vi "AIT 1553 System Definition API Example.vi"() -> ()   [LabVIEW 2011]
uses:
  Controls/AIT 1553 Settings.ctl
  System Explorer/Controls/1553 Bus Enabled.ctl
  NationalInstruments.VeriStand.SystemDefinitionAPI
  AIT 1553 Custom Device.lvlib
panel:
  out "error":string
  out "error out":errorcluster
  in  "error in (no error)":errorcluster
  out "Sysdef Path":path=path "C:/Users/Public/Documents/National Instruments/NI VeriStand 2011/Projects/DynamicallyCreatedProject/DynamicallyCreatedProject.nivssdf"
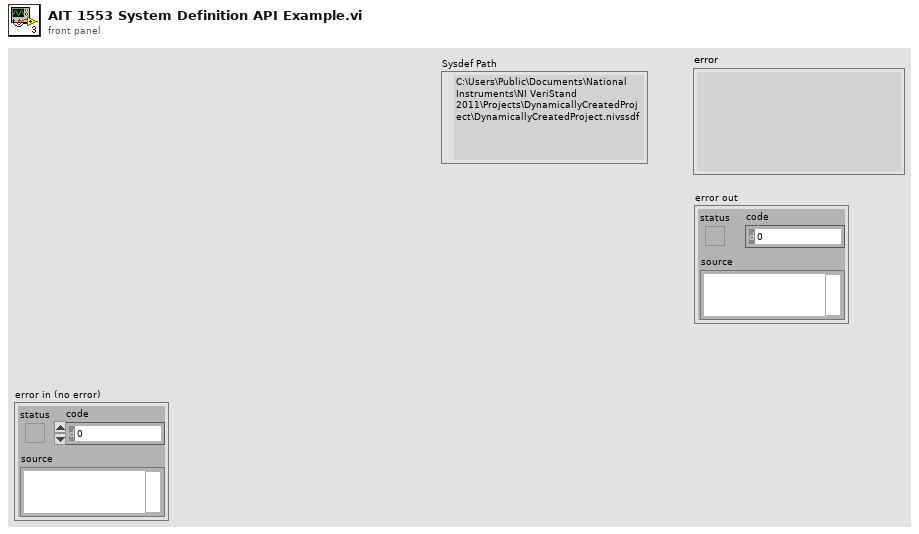
[diagram p1: front panel]
types:
  T1 = typedef "AIT 1553 Settings.ctl" = cluster{"Board Serial #":u64, "AppLicense":bool, "License Key":string, "BusEnabledProperties":T2, "Description":string, "Bus1 Path":path, "Bus2 Path":path, "Bus3 Path":path, "Bus4 Path":path}
  T2 = typedef "AIT 1553 Custom Device.lvlib/1553 Bus Enabled.ctl" = cluster{"Bus1Enabled":bool, "Bus2Enabled":bool, "Bus3Enabled":bool, "Bus4Enabled":bool}
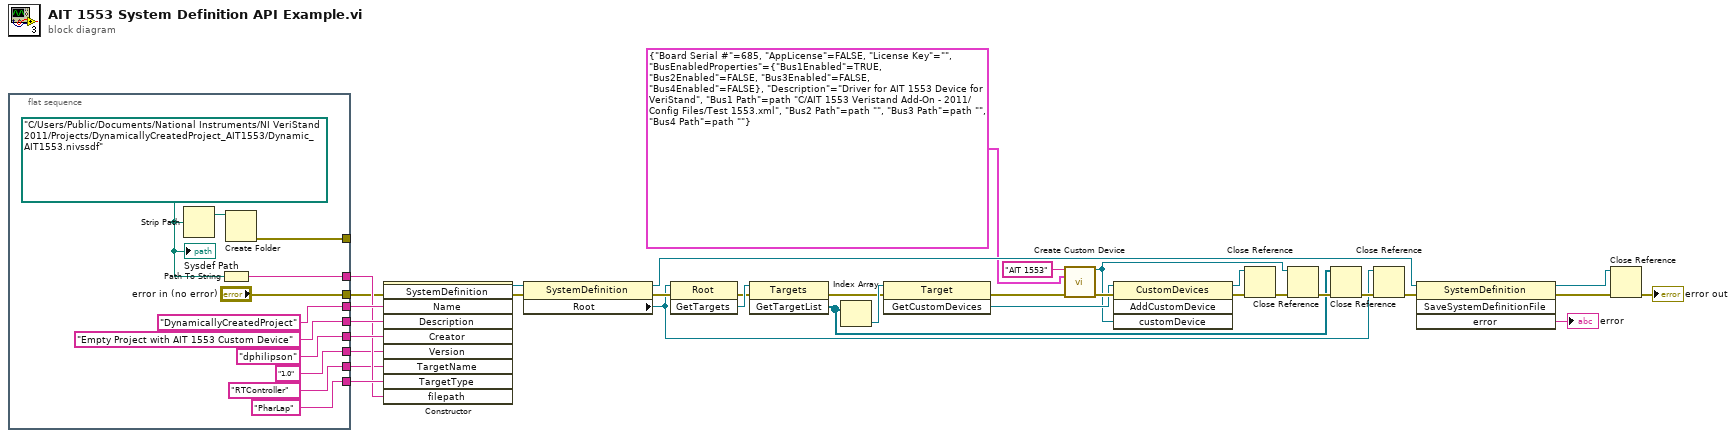
[diagram p0: block diagram]
diagram:
  n1 = flat-sequence {
    tunnel: ["DynamicallyCreatedProject" ("Name")] -> w34
    tunnel: ["dphilipson" ("Creator")] -> w33
    tunnel: ["RTController" ("TargetName")] -> w23
    tunnel: ["PharLap" ("TargetType")] -> w32
    tunnel: ["Empty Project with AIT 1553 Custom Device" ("Description")] -> w31
    tunnel: [w38] -> w30
    tunnel: [w37] -> _
    tunnel: ["error in (no error)"] -> w24
    tunnel: ["1.0" ("Version")] -> w22
    frame #0 {
      w39 = path "C:/Users/Public/Documents/National Instruments/NI VeriStand 2011/Projects/DynamicallyCreatedProject_AIT1553/Dynamic_AIT1553.nivssdf"
      n2 = Strip Path(path=w39) -> (stripped path=w40:path)  [unwired: 1 out]
      n3 = Path To String(path=w39) -> (string=w38:string)
      n4 = Create Folder(path (use dialog)=w40) -> (error out=w37:errorcluster)  [unwired: 2 in, 2 out]
      "Sysdef Path" <- w39
    }
  }
  n5 = constructor class="SystemDefinition"(error in=w24, "Name"=w34, "Description"=w31, "Creator"=w33, "Version"=w22, "TargetName"=w23, "TargetType"=w32, "filepath"=w30) -> (reference out=w26:refnum<k24>, error out=w28:errorcluster)  [unwired: 2 in, 8 out]
  n6 = property class="SystemDefinition"(reference=w26, error in=w28) -> (reference out=w13:refnum<k24>, error out=w27:errorcluster, "Root"=w12:refnum<k24>)
  n7 = invoke class="Root" method="GetTargets"(reference=w12, error in=w27) -> (error out=w25:errorcluster, "GetTargets"=w29:refnum<k24>)  [unwired: 1 in, 1 out]
  n8 = invoke class="Targets" method="GetTargetList"(reference=w29, error in=w25) -> (error out=w14:errorcluster, "GetTargetList"=w11:refnum<k24>[])  [unwired: 1 in, 1 out]
  n9 = Index Array(array=w11) -> (element=w15:refnum<k24>)  [unwired: 1 in]
  n10 = invoke class="Target" method="GetCustomDevices"(reference=w15, error in=w14) -> (error out=w10:errorcluster, "GetCustomDevices"=w5:refnum<k24>)  [unwired: 1 in, 1 out]
  n11 = call "Create Custom Device.vi"("Name"="AIT 1553", "AIT 1553 Settings"=T1 {"Board Serial #"=685, "AppLicense"=FALSE, "License Key"="", "BusEnabledProperties"={"Bus1Enabled"=TRUE, "Bus2Enabled"=FALSE, "Bus3Enabled"=FALSE, "Bus4Enabled"=FALSE}, "Description"="Driver for AIT 1553 Device for VeriStand", "Bus1 Path"=path "C:/AIT 1553 Veristand Add-On - 2011/Config Files/Test 1553.xml", "Bus2 Path"=path "", "Bus3 Path"=path "", "Bus4 Path"=path ""}, "error in (no error)"=w10) -> ("Custom Device reference"=w1:refnum<k24>, "error out"=w9:errorcluster)  [unwired: 11 in]
  n12 = invoke class="CustomDevices" method="AddCustomDevice"(reference=w5, error in=w9, "customDevice"=w1) -> (reference out=w4:refnum<k24>, error out=w2:errorcluster)  [unwired: 1 in, 2 out]
  n13 = Close Reference(reference=w4, error in (no error)=w2) -> (error out=w3:errorcluster)
  n14 = Close Reference(reference=w1, error in (no error)=w3) -> (error out=w16:errorcluster)
  n15 = Close Reference(reference=w11, error in (no error)=w16) -> (error out=w18:errorcluster)
  n16 = Close Reference(reference=w12, error in (no error)=w18) -> (error out=w17:errorcluster)
  n17 = invoke class="SystemDefinition" method="SaveSystemDefinitionFile"(reference=w13, error in=w17) -> (reference out=w19:refnum<k24>, error out=w21:errorcluster, "error"=→"error":string)  [unwired: 2 in, 1 out]
  n18 = Close Reference(reference=w19, error in (no error)=w21) -> (error out=→"error out":errorcluster)
